vi "WinnersTicTacToe_Final.vi"() -> ()   [LabVIEW 2024]
panel:
  out "RULES":string
  out "INSTRUCTIONS":string
  out "GAME OVER":string
  in  "CLEAR":bool
  out "Turn":string
  in  "Set Player Turn":bool
  in  "BR":bool
  in  "BM":bool
  in  "BL":bool
  in  "MR":bool
  in  "MM":bool
  in  "ML":bool
  in  "UR":bool
  in  "UM":bool
  in  "UL":bool
  in  "START/END":bool
  in  "EXIT BUTTON":bool
  out "Title":string="TIC TAC TOE GAME"
  out "\"Player 1\"":string="Player 1"
  out "\"Player 2\"":string="Player 2"
  out "String \"X\"":string="X"
  out "String \"O\"":string="O"
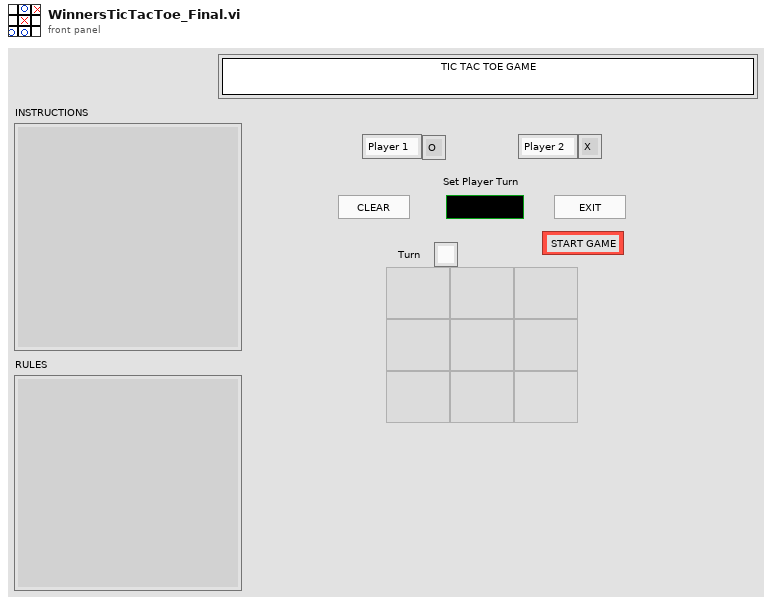
[diagram p1: front panel]
types:
  T1 = enum8{"Enabled", "Disabled", "Disabled and Grayed Out"}
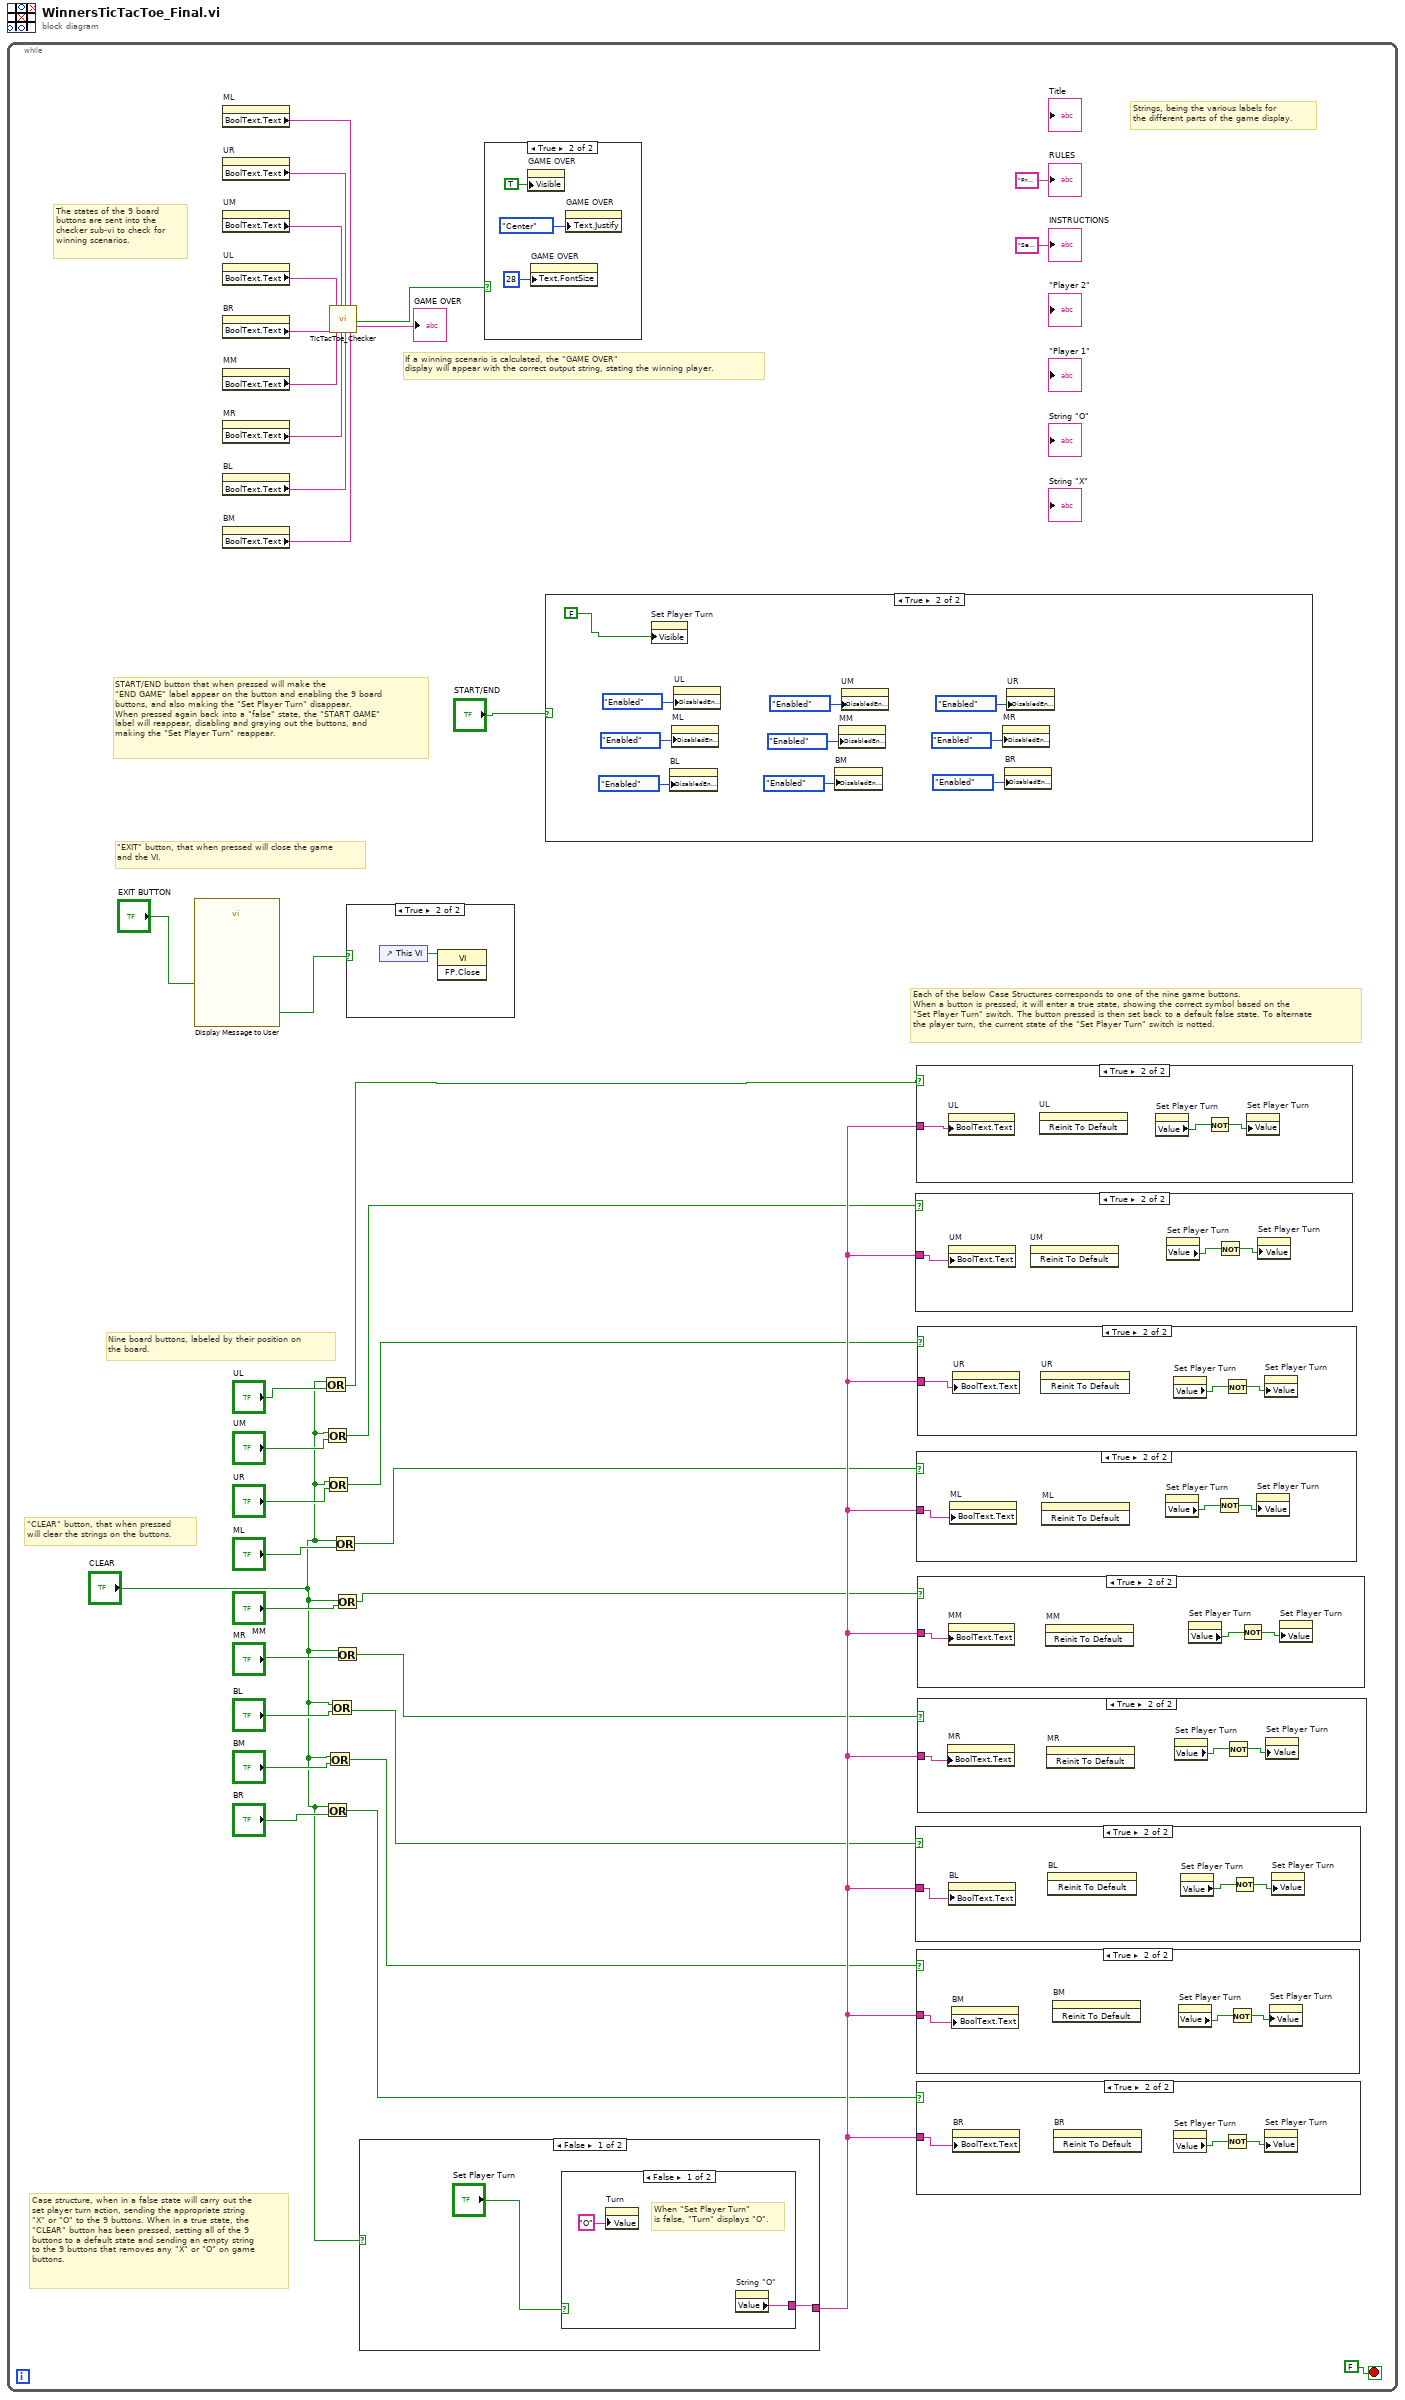
[diagram p0: block diagram]
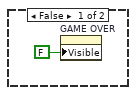
[diagram p2: hidden frame]
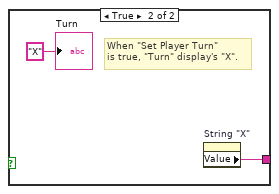
[diagram p3: hidden frame]
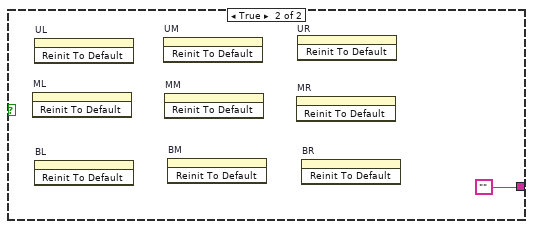
[diagram p4: hidden frame]
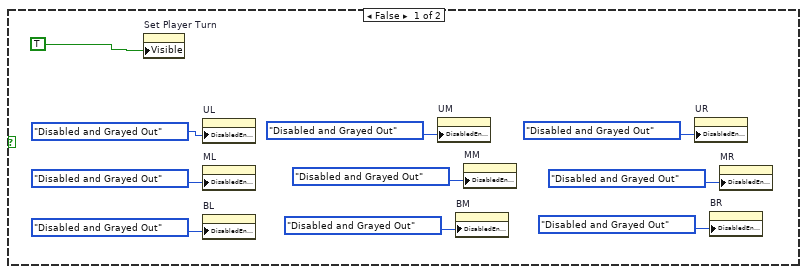
[diagram p5: hidden frame]
diagram:
  n1 = while {
    stop <- FALSE stop-if-true
    # "Each of the below Case Structures corresponds to one of the nine game buttons.\nWhen a button is pressed, it will enter a true state, showing the correct symbol based on the \n\"Set Player Turn\" switch. The button pressed is then set back to a default false state. To alternate\nthe player turn, the current state of the \"Set Player Turn\" switch is notted."
    # "Case structure, when in a false state will carry out the\nset player turn action, sending the appropriate string\n\"X\" or \"O\" to the 9 buttons. When in a true state, the \n\"CLEAR\" button has been pressed, setting all of the 9\nbuttons to a default state and sending an empty string\nto the 9 buttons that removes any \"X\" or \"O\" on game\nbuttons."
    # "\"CLEAR\" button, that when pressed\nwill clear the strings on the buttons."
    # "Nine board buttons, labeled by their position on\nthe board."
    # "\"EXIT\" button, that when pressed will close the game\nand the VI."
    # "START/END button that when pressed will make the \n\"END GAME\" label appear on the button and enabling the 9 board \nbuttons, and also making the \"Set Player Turn\" disappear. \nWhen pressed again back into a \"false\" state, the \"START GAME\"\nlabel will reappear, disabling and graying out the buttons, and\nmaking the \"Set Player Turn\" reappear."
    # "If a winning scenario is calculated, the \"GAME OVER\" \ndisplay will appear with the correct output string, stating the winning player."
    # "The states of the 9 board \nbuttons are sent into the \nchecker sub-vi to check for \nwinning scenarios."
    # "Strings, being the various labels for\nthe different parts of the game display."
    n2 = call "Display Message to User"("Enable"="EXIT BUTTON") -> ("EXIT"=w36:bool)  [unwired: 9 in, 1 out]
    n3 = property on="ML" class="Bool (strict)"() -> ("BoolText.Text"=w10:string)  [unwired: 2 in, 2 out]
    n4 = property on="UR" class="Bool (strict)"() -> ("BoolText.Text"=w11:string)  [unwired: 2 in, 2 out]
    n5 = property on="UM" class="Bool (strict)"() -> ("BoolText.Text"=w12:string)  [unwired: 2 in, 2 out]
    n6 = property on="UL" class="Bool (strict)"() -> ("BoolText.Text"=w13:string)  [unwired: 2 in, 2 out]
    n7 = property on="BR" class="Bool (strict)"() -> ("BoolText.Text"=w5:string)  [unwired: 2 in, 2 out]
    n8 = property on="MM" class="Bool (strict)"() -> ("BoolText.Text"=w9:string)  [unwired: 2 in, 2 out]
    n9 = property on="MR" class="Bool (strict)"() -> ("BoolText.Text"=w8:string)  [unwired: 2 in, 2 out]
    n10 = property on="BL" class="Bool (strict)"() -> ("BoolText.Text"=w7:string)  [unwired: 2 in, 2 out]
    n11 = property on="BM" class="Bool (strict)"() -> ("BoolText.Text"=w6:string)  [unwired: 2 in, 2 out]
    n12 = Or(x="CLEAR", y="UL") -> (x .or. y?=w3:bool)
    n13 = Or(x="CLEAR", y="UM") -> (x .or. y?=w31:bool)
    n14 = Or(x="CLEAR", y="BR") -> (x .or. y?=w16:bool)
    n15 = Or(x="CLEAR", y="UR") -> (x .or. y?=w29:bool)
    n16 = Or(x="CLEAR", y="BM") -> (x .or. y?=w19:bool)
    n17 = Or(x="CLEAR", y="BL") -> (x .or. y?=w21:bool)
    n18 = call "TicTacToe_Checker.vi"("BR"=w5, "UL"=w13, "MM"=w9, "UM"=w12, "MR"=w8, "UR"=w11, "BL"=w7, "ML"=w10, "BM"=w6) -> ("P1 or P2?"=w4:bool, "\"GAME OVER\""=→"GAME OVER":string)  [unwired: 9 in]
    n19 = Or(x="CLEAR", y="ML") -> (x .or. y?=w27:bool)
    n20 = Or(x="CLEAR", y="MM") -> (x .or. y?=w25:bool)
    n21 = Or(x="CLEAR", y="MR") -> (x .or. y?=w23:bool)
    n22 = case shown="True" w36 {
      frame False {
      }
      frame True {
        n23 = control-ref of="This VI"() -> (w69:refnum<vi>)
        n24 = invoke class="VI" method="FP.Close"(reference=w69) -> ()  [unwired: 2 in, 3 out]
      }
    }
    n25 = case shown="False" "CLEAR" {
      tunnel: [w42 ""] -> w33
      frame False {
        n26 = case shown="False" "Set Player Turn" {
          tunnel: [w44 w46] -> w42
          frame False {
            # "When \"Set Player Turn\"\nis false, \"Turn\" displays \"O\"."
            n27 = property on="Turn" class="Str"("Value"="O" ("Current Symbol 2")) -> ()  [unwired: 2 in, 2 out]
            n28 = property on="String \"O\"" class="Str"() -> ("Value"=w44:string)  [unwired: 2 in, 2 out]
          }
          frame True {
            # "When \"Set Player Turn\"\nis true, \"Turn\" display's \"X\"."
            n29 = property on="String \"X\"" class="Str"() -> ("Value"=w46:string)  [unwired: 2 in, 2 out]
            "Turn" <- "X" ("Current Symbol")
          }
        }
      }
      frame True {
        n30 = invoke on="ML" class="Bool (strict)" method="Reinit To Default"() -> ()  [unwired: 3 in, 3 out]
        n31 = invoke on="UL" class="Bool (strict)" method="Reinit To Default"() -> ()  [unwired: 3 in, 3 out]
        n32 = invoke on="BL" class="Bool (strict)" method="Reinit To Default"() -> ()  [unwired: 3 in, 3 out]
        n33 = invoke on="UM" class="Bool (strict)" method="Reinit To Default"() -> ()  [unwired: 3 in, 3 out]
        n34 = invoke on="MM" class="Bool (strict)" method="Reinit To Default"() -> ()  [unwired: 3 in, 3 out]
        n35 = invoke on="BM" class="Bool (strict)" method="Reinit To Default"() -> ()  [unwired: 3 in, 3 out]
        n36 = invoke on="MR" class="Bool (strict)" method="Reinit To Default"() -> ()  [unwired: 3 in, 3 out]
        n37 = invoke on="UR" class="Bool (strict)" method="Reinit To Default"() -> ()  [unwired: 3 in, 3 out]
        n38 = invoke on="BR" class="Bool (strict)" method="Reinit To Default"() -> ()  [unwired: 3 in, 3 out]
      }
    }
    n39 = case shown="True" w4 {
      frame False {
        n40 = property on="GAME OVER" class="Str"("Visible"=FALSE) -> ()  [unwired: 2 in, 2 out]
      }
      frame True {
        n41 = property on="GAME OVER" class="Str"("Visible"=TRUE) -> ()  [unwired: 2 in, 2 out]
        n42 = property on="GAME OVER" class="Str"("Text.FontSize"=u32 28 ("Text.Font:Size")) -> ()  [unwired: 2 in, 2 out]
        n43 = property on="GAME OVER" class="Str"("Text.Justify"=enum16{"Left", "Center", "Right"}."Center" ("Text.Justification")) -> ()  [unwired: 2 in, 2 out]
      }
    }
    n44 = case shown="True" "START/END" {
      frame False {
        n45 = property on="Set Player Turn" class="Bool (strict)"("Visible"=TRUE) -> ()  [unwired: 2 in, 2 out]
        n46 = property on="UL" class="Bool (strict)"("DisabledEnum"=T1."Disabled and Grayed Out" ("Disabled")) -> ()  [unwired: 2 in, 2 out]
        n47 = property on="ML" class="Bool (strict)"("DisabledEnum"=T1."Disabled and Grayed Out" ("Disabled")) -> ()  [unwired: 2 in, 2 out]
        n48 = property on="BL" class="Bool (strict)"("DisabledEnum"=T1."Disabled and Grayed Out" ("Disabled")) -> ()  [unwired: 2 in, 2 out]
        n49 = property on="UM" class="Bool (strict)"("DisabledEnum"=T1."Disabled and Grayed Out" ("Disabled")) -> ()  [unwired: 2 in, 2 out]
        n50 = property on="BM" class="Bool (strict)"("DisabledEnum"=T1."Disabled and Grayed Out" ("Disabled")) -> ()  [unwired: 2 in, 2 out]
        n51 = property on="MM" class="Bool (strict)"("DisabledEnum"=T1."Disabled and Grayed Out" ("Disabled")) -> ()  [unwired: 2 in, 2 out]
        n52 = property on="UR" class="Bool (strict)"("DisabledEnum"=T1."Disabled and Grayed Out" ("Disabled")) -> ()  [unwired: 2 in, 2 out]
        n53 = property on="BR" class="Bool (strict)"("DisabledEnum"=T1."Disabled and Grayed Out" ("Disabled")) -> ()  [unwired: 2 in, 2 out]
        n54 = property on="MR" class="Bool (strict)"("DisabledEnum"=T1."Disabled and Grayed Out" ("Disabled")) -> ()  [unwired: 2 in, 2 out]
      }
      frame True {
        n55 = property on="Set Player Turn" class="Bool (strict)"("Visible"=FALSE) -> ()  [unwired: 2 in, 2 out]
        n56 = property on="BL" class="Bool (strict)"("DisabledEnum"=T1."Enabled" ("Disabled")) -> ()  [unwired: 2 in, 2 out]
        n57 = property on="ML" class="Bool (strict)"("DisabledEnum"=T1."Enabled" ("Disabled")) -> ()  [unwired: 2 in, 2 out]
        n58 = property on="UL" class="Bool (strict)"("DisabledEnum"=T1."Enabled" ("Disabled")) -> ()  [unwired: 2 in, 2 out]
        n59 = property on="BM" class="Bool (strict)"("DisabledEnum"=T1."Enabled" ("Disabled")) -> ()  [unwired: 2 in, 2 out]
        n60 = property on="MM" class="Bool (strict)"("DisabledEnum"=T1."Enabled" ("Disabled")) -> ()  [unwired: 2 in, 2 out]
        n61 = property on="UM" class="Bool (strict)"("DisabledEnum"=T1."Enabled" ("Disabled")) -> ()  [unwired: 2 in, 2 out]
        n62 = property on="MR" class="Bool (strict)"("DisabledEnum"=T1."Enabled" ("Disabled")) -> ()  [unwired: 2 in, 2 out]
        n63 = property on="BR" class="Bool (strict)"("DisabledEnum"=T1."Enabled" ("Disabled")) -> ()  [unwired: 2 in, 2 out]
        n64 = property on="UR" class="Bool (strict)"("DisabledEnum"=T1."Enabled" ("Disabled")) -> ()  [unwired: 2 in, 2 out]
      }
    }
    n65 = case shown="True" w31 {
      tunnel: w33 -> [_ w75]
      frame False {
      }
      frame True {
        n66 = property on="UM" class="Bool (strict)"("BoolText.Text"=w75) -> ()  [unwired: 2 in, 2 out]
        n67 = invoke on="UM" class="Bool (strict)" method="Reinit To Default"() -> ()  [unwired: 3 in, 3 out]
        n68 = property on="Set Player Turn" class="Bool (strict)"() -> ("Value"=w74:bool)  [unwired: 2 in, 2 out]
        n69 = Not(x=w74) -> (.not. x?=w73:bool)
        n70 = property on="Set Player Turn" class="Bool (strict)"("Value"=w73) -> ()  [unwired: 2 in, 2 out]
      }
    }
    n71 = case shown="True" w21 {
      tunnel: w33 -> [_ w84]
      frame False {
      }
      frame True {
        n72 = property on="BL" class="Bool (strict)"("BoolText.Text"=w84) -> ()  [unwired: 2 in, 2 out]
        n73 = invoke on="BL" class="Bool (strict)" method="Reinit To Default"() -> ()  [unwired: 3 in, 3 out]
        n74 = property on="Set Player Turn" class="Bool (strict)"() -> ("Value"=w83:bool)  [unwired: 2 in, 2 out]
        n75 = Not(x=w83) -> (.not. x?=w82:bool)
        n76 = property on="Set Player Turn" class="Bool (strict)"("Value"=w82) -> ()  [unwired: 2 in, 2 out]
      }
    }
    n77 = case shown="True" w3 {
      tunnel: w33 -> [_ w78]
      frame False {
      }
      frame True {
        n78 = property on="UL" class="Bool (strict)"("BoolText.Text"=w78) -> ()  [unwired: 2 in, 2 out]
        n79 = invoke on="UL" class="Bool (strict)" method="Reinit To Default"() -> ()  [unwired: 3 in, 3 out]
        n80 = property on="Set Player Turn" class="Bool (strict)"() -> ("Value"=w77:bool)  [unwired: 2 in, 2 out]
        n81 = Not(x=w77) -> (.not. x?=w76:bool)
        n82 = property on="Set Player Turn" class="Bool (strict)"("Value"=w76) -> ()  [unwired: 2 in, 2 out]
      }
    }
    n83 = case shown="True" w27 {
      tunnel: w33 -> [_ w93]
      frame False {
      }
      frame True {
        n84 = property on="ML" class="Bool (strict)"("BoolText.Text"=w93) -> ()  [unwired: 2 in, 2 out]
        n85 = invoke on="ML" class="Bool (strict)" method="Reinit To Default"() -> ()  [unwired: 3 in, 3 out]
        n86 = property on="Set Player Turn" class="Bool (strict)"() -> ("Value"=w92:bool)  [unwired: 2 in, 2 out]
        n87 = Not(x=w92) -> (.not. x?=w91:bool)
        n88 = property on="Set Player Turn" class="Bool (strict)"("Value"=w91) -> ()  [unwired: 2 in, 2 out]
      }
    }
    n89 = case shown="True" w19 {
      tunnel: w33 -> [_ w72]
      frame False {
      }
      frame True {
        n90 = property on="BM" class="Bool (strict)"("BoolText.Text"=w72) -> ()  [unwired: 2 in, 2 out]
        n91 = invoke on="BM" class="Bool (strict)" method="Reinit To Default"() -> ()  [unwired: 3 in, 3 out]
        n92 = property on="Set Player Turn" class="Bool (strict)"() -> ("Value"=w71:bool)  [unwired: 2 in, 2 out]
        n93 = Not(x=w71) -> (.not. x?=w70:bool)
        n94 = property on="Set Player Turn" class="Bool (strict)"("Value"=w70) -> ()  [unwired: 2 in, 2 out]
      }
    }
    n95 = case shown="True" w16 {
      tunnel: w33 -> [_ w81]
      frame False {
      }
      frame True {
        n96 = property on="BR" class="Bool (strict)"("BoolText.Text"=w81) -> ()  [unwired: 2 in, 2 out]
        n97 = invoke on="BR" class="Bool (strict)" method="Reinit To Default"() -> ()  [unwired: 3 in, 3 out]
        n98 = property on="Set Player Turn" class="Bool (strict)"() -> ("Value"=w80:bool)  [unwired: 2 in, 2 out]
        n99 = Not(x=w80) -> (.not. x?=w79:bool)
        n100 = property on="Set Player Turn" class="Bool (strict)"("Value"=w79) -> ()  [unwired: 2 in, 2 out]
      }
    }
    n101 = case shown="True" w29 {
      tunnel: w33 -> [_ w96]
      frame False {
      }
      frame True {
        n102 = property on="UR" class="Bool (strict)"("BoolText.Text"=w96) -> ()  [unwired: 2 in, 2 out]
        n103 = invoke on="UR" class="Bool (strict)" method="Reinit To Default"() -> ()  [unwired: 3 in, 3 out]
        n104 = property on="Set Player Turn" class="Bool (strict)"() -> ("Value"=w95:bool)  [unwired: 2 in, 2 out]
        n105 = Not(x=w95) -> (.not. x?=w94:bool)
        n106 = property on="Set Player Turn" class="Bool (strict)"("Value"=w94) -> ()  [unwired: 2 in, 2 out]
      }
    }
    n107 = case shown="True" w25 {
      tunnel: w33 -> [_ w90]
      frame False {
      }
      frame True {
        n108 = property on="MM" class="Bool (strict)"("BoolText.Text"=w90) -> ()  [unwired: 2 in, 2 out]
        n109 = invoke on="MM" class="Bool (strict)" method="Reinit To Default"() -> ()  [unwired: 3 in, 3 out]
        n110 = property on="Set Player Turn" class="Bool (strict)"() -> ("Value"=w89:bool)  [unwired: 2 in, 2 out]
        n111 = Not(x=w89) -> (.not. x?=w88:bool)
        n112 = property on="Set Player Turn" class="Bool (strict)"("Value"=w88) -> ()  [unwired: 2 in, 2 out]
      }
    }
    n113 = case shown="True" w23 {
      tunnel: w33 -> [_ w87]
      frame False {
      }
      frame True {
        n114 = property on="MR" class="Bool (strict)"("BoolText.Text"=w87) -> ()  [unwired: 2 in, 2 out]
        n115 = invoke on="MR" class="Bool (strict)" method="Reinit To Default"() -> ()  [unwired: 3 in, 3 out]
        n116 = property on="Set Player Turn" class="Bool (strict)"() -> ("Value"=w86:bool)  [unwired: 2 in, 2 out]
        n117 = Not(x=w86) -> (.not. x?=w85:bool)
        n118 = property on="Set Player Turn" class="Bool (strict)"("Value"=w85) -> ()  [unwired: 2 in, 2 out]
      }
    }
    "INSTRUCTIONS" <- "Set Player Turn: Set switch to change starting player.\n\nStart Game: Press to begin the match.\n\nTurn: Shows the current player's turn.\n\nEnd Game: Press to end the match.\n\nClear: Press to remove all symbols from the board.\n\nExit: Press to close the program."
    "RULES" <- "Press a box to place the symbol of the player with the active turn.\n\nPlayers can \"steal\" a box from the other by placing their symbol on\na box where the other player's symbol already resides.\n\nA player wins the game when they get three of their symbol in a row.\n\nThere is ALWAYS a winner, this game can't end in a tie."
  }
